vi "LaunchServerGUI.vi"(8 "error in (no error)":errorcluster, 11 "TCP_Server in":refnum<class "TCP_Server.lvclass">) -> (0 "error out":errorcluster, 3 "TCP_Server out":refnum<class "TCP_Server.lvclass">)   [LabVIEW 2023, in "TCP_Server.lvlib" / "TCP_Server.lvclass"]
uses:
  TCP_Server.lvclass
  TCP_Server.lvclass/TCP_Server.ctl
  <vilib>/ActorFramework/Actor/Actor.lvclass
  TCP_serverGUI/TCP_serverGUI/TCP_serverGUI.lvclass
  TCP_serverGUI/TCP_serverGUI Messages/UpdateServerAddress Msg/UpdateServerAddress Msg.lvclass
  C:/Program Files (x86)/National Instruments/LabVIEW 2023/vi.lib/ActorFramework/Actor/Actor.lvclass
  C:/Source/LabVIEW/TCP_server/TCP_serverGUI/TCP_serverGUI/TCP_serverGUI.lvclass
  C:/Source/LabVIEW/TCP_server/TCP_Server/TCP_Server/TCP_Server.lvclass
  C:/Source/LabVIEW/TCP_server/SimpleErrorLogger/ApplicationWithErrorLogger/ApplicationWithErrorLogger.lvclass
  C:/Source/LabVIEW/TCP_server/TCP_Client_Window/TCP_ClientWindow_Controller/TCP_ClientWindow_Controller.lvclass
  C:/Source/LabVIEW/TCP_server/TCP_Listener/Connections Controller/Connections Controller.lvclass
  C:/Source/LabVIEW/TCP_server/TCP_Server_Connection_Handler/TCP_Connections_Controller/TCP_Connections_Controller.lvclass
  C:/Source/LabVIEW/TCP_server/TCP_serverGUI/TCP_ServerWithGUI/TCP_ServerWithGUI.lvclass
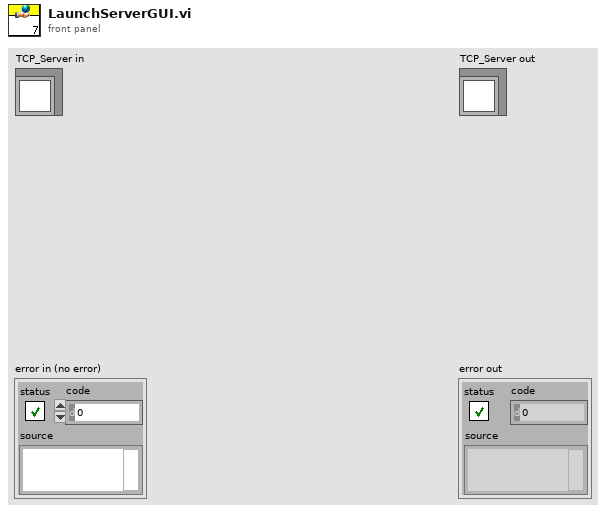
[diagram p1: front panel]
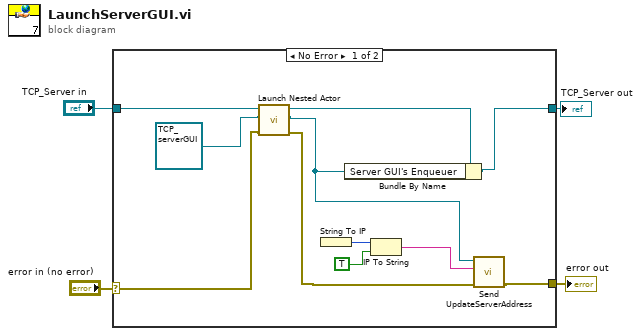
[diagram p0: block diagram]
diagram:
  n1 = case shown="No Error" "error in (no error)" {
    selector: "error in (no error)" -> [w13 w17]
    tunnel: [w5 w17] -> w3
    tunnel: [w6 w16] -> w1
    tunnel: "TCP_Server in" -> [w15 w16]
    frame No Error {
      n2 = call <vilib>:"Launch Nested Actor.vi"("error in (no error)"=w13, "Nested Actor"=refnum<class "TCP_serverGUI.lvclass"> refnum ("TCP_serverGUI.lvlib:TCP_serverGUI.lvclass"), "Caller Actor in"=w15) -> ("error out"=w7:errorcluster, "Nested Actor's Enqueuer"=w11:refnum<class "Message Enqueuer.lvclass">, "Caller Actor out"=w12:refnum<class "TCP_Server.lvclass">)  [unwired: 6 in]
      n3 = String To IP() -> (0:w10:u32)  [unwired: 1 in]
      n4 = Bundle By Name(cluster=w12, "Server GUI's Enqueuer"=w11) -> (w6:refnum<class "TCP_Server.lvclass">)
      n5 = IP To String(1:TRUE ("dot notation? (F)"), 2:w10) -> (0:w8:string)
      n6 = call "Send UpdateServerAddress.vi"("error in (no error)"=w7, "Server address"=w8, "Message Enqueuer"=w11) -> ("error out"=w5:errorcluster)  [unwired: 7 in, 1 out]
    }
    frame Error {
    }
  }
  "error out" <- w3
  "TCP_Server out" <- w1
